vi "GMU2 Calib Shutdown.vi"() -> ()   [LabVIEW 2022 SP3]
uses:
  Traverse_cluster.ctl
  Spacing.ctl
  Controls/Multi_run_mode.ctl
  Controls/User_Specific_mode.ctl
  ADAM Client/Sub VIs/ADAM Controls/Client_Source_Status.ctl
  Controls/GMU Gas Line Name.ctl
panel:
  in  "stop":bool
  out "Purge time (s)":sgl(slide) scale=0.0..600.0
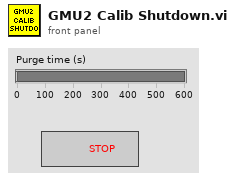
[diagram p1: front panel]
types:
  T1 = typedef "GMU Gas Line Name.ctl" = enum16{"GMU1 Source", "GMU2 Source", "GMU2 Calib", "CPP GRC-A", "CPP GRC-B"}
  T2 = typedef "Client_Source_Status.ctl" = enum16{"Not Using", "Using", "Must Have"}
  T3 = typedef "User_Specific_mode.ctl" = enum16{"Check VI only", "Run VI"}
  T4 = typedef "Traverse_cluster.ctl" = cluster{"Start X":sgl, "Start Y":sgl, "Start Z":sgl, "End X":sgl, "End Y":sgl, "End Z":sgl, "nPoints":i32, "Spacing":T5, "Filename":path, "Tunnel Speed":dbl, "Averaging time (mins)":dbl, "Extra Commands":string, "Carrier_1 Q (l/min)":dbl, "Carrier_2 Q (l/min)":dbl, "Trace Gas Concentration (%)":dbl, "Specific Arguments":string, "Comments":string, "Row No":i32, "Row Type Selector":T6, "EstCompl":string, "Row Duration (mins)":dbl, "nValidPoints":i32, "Meas Setup File":string}
  T5 = typedef "Spacing.ctl" = enum16{"Linear", "Log", "Gauss", "Specified", "N/A"}
  T6 = typedef "Multi_run_mode.ctl" = enum16{"Move Traverse Only", "Set Tunnel Speed Only", "Set Source Only", "Set Measurement Conditions", "Single Measurement", "Vertical Profile", "Lateral Profile", "Longitudinal Profile", "Multi-Axis Profile", "Explore Volume", "Auto Calibrate", "Meas Fast FID Bkgnd", "Check Beam Power", "Scanning Valve Measurement", "Run VI Named:", "Set ADAM Ch", "Wait (minutes)", "Send Message", "Synchronize With:", "Fall Back to this Row", "Turn Off Row Repeating", "Traverse 3D Volume", "Blank Row", "Jump to Fall Back Row"}
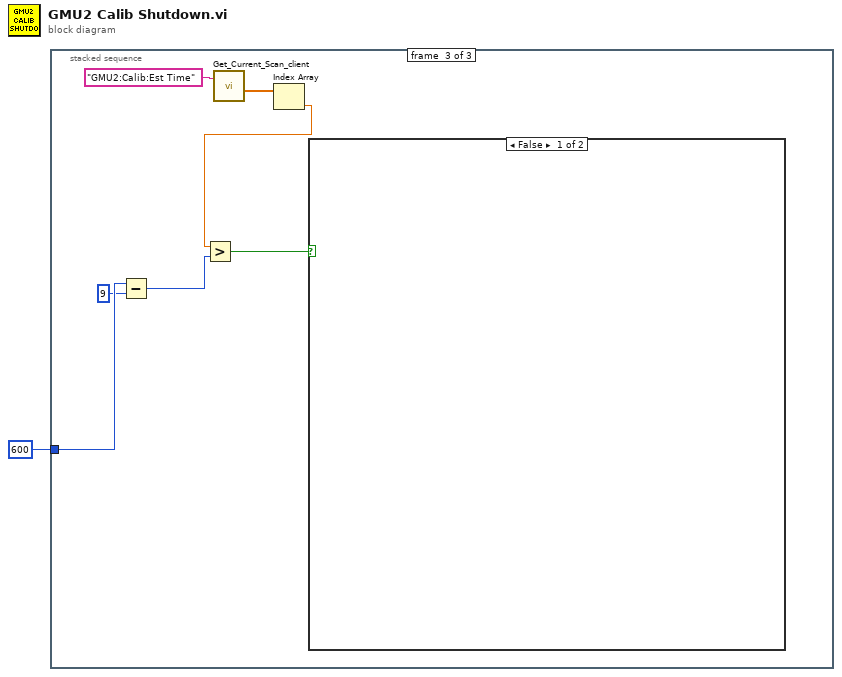
[diagram p0: block diagram]
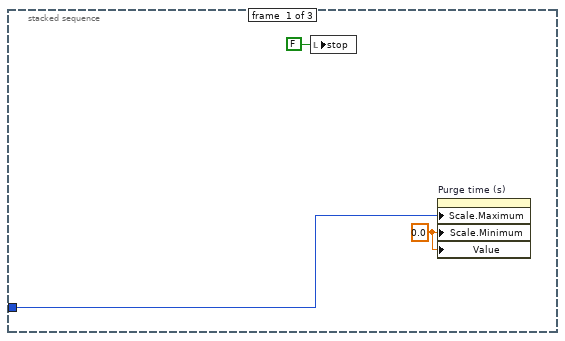
[diagram p2: hidden frame]
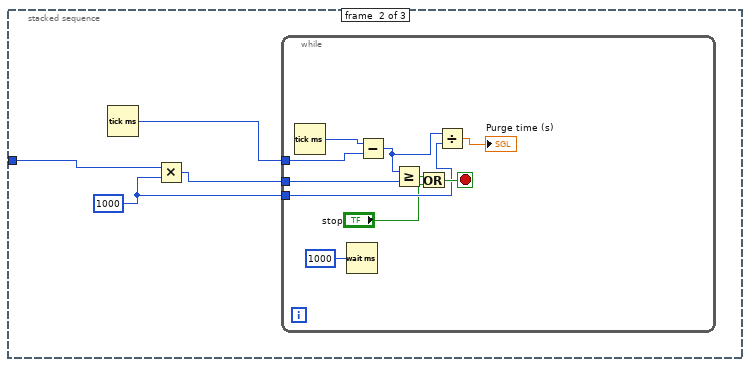
[diagram p3: hidden frame]
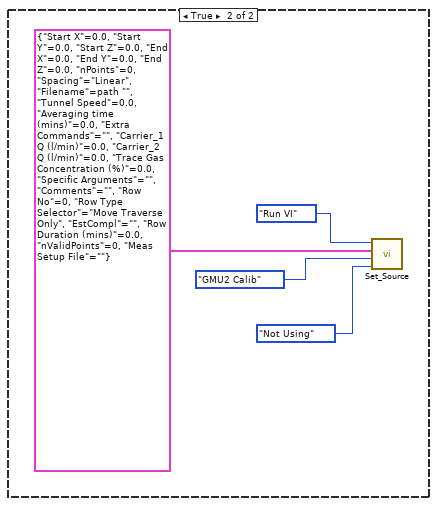
[diagram p4: hidden frame]
diagram:
  n1 = stacked-sequence {
    tunnel: 600 -> [w4 w7 w22]
    frame #0 {
      w3 = 0.0 ("Scale.Range:Minimum")
      n2 = local write "stop"(FALSE ("stop")) -> ()
      n3 = property on="Purge time (s)" class="Slide (strict)"("Scale.Maximum"=w4, "Scale.Minimum"=w3, "Value"=w3) -> ()  [unwired: 2 in, 2 out]
    }
    frame #1 {
      w5 = 1000 ("y")
      n4 = Tick Count (ms)() -> (millisecond timer value=w8:u32)
      n5 = Multiply(x=w7, y=w5) -> (x*y=w6:i32)
      n6 = while {
        tunnel: w6 -> [w17]
        tunnel: w8 -> [w13]
        tunnel: w5 -> [w11]
        stop <- w15 stop-if-true
        n7 = Tick Count (ms)() -> (millisecond timer value=w14:u32)
        n8 = Wait (ms)(milliseconds to wait=u32 1000) -> ()  [unwired: 1 out]
        n9 = Subtract(x=w14, y=w13) -> (x-y=w12:u32)
        n10 = Greater Or Equal?(x=w12, y=w17) -> (x >= y?=w16:bool)
        n11 = Or(x=w16, y="stop") -> (x .or. y?=w15:bool)
        n12 = Divide(x=w12, y=w11) -> (x/y=→"Purge time (s)":dbl)
      }
    }
    frame #2 {
      n13 = Subtract(x=w22, y=9) -> (x-y=w20:i32)
      n14 = call "Get_Current_Scan_client.vi"("singleChannel"="GMU2:Calib:Est Time") -> ("Numerical Values"=w25:dbl[])  [unwired: 1 in, 3 out]
      n15 = Index Array(array=w25) -> (element=w23:dbl)  [unwired: 1 in]
      n16 = Greater?(x=w23, y=w20) -> (0:w19:bool)
      n17 = case shown="False" w19 {
        frame False {
        }
        frame True {
          n18 = call "Set_Source.vi"("Source Status"=Client_Source_Status."Not Using", "Gas Line Name"=GMU_Gas_Line_Name."GMU2 Calib", "Traverse line"=T4 {"Start X"=0.0, "Start Y"=0.0, "Start Z"=0.0, "End X"=0.0, "End Y"=0.0, "End Z"=0.0, "nPoints"=0, "Spacing"=enum."Linear", "Filename"=path "", "Tunnel Speed"=0.0, "Averaging time (mins)"=0.0, "Extra Commands"="", "Carrier_1 Q (l/min)"=0.0, "Carrier_2 Q (l/min)"=0.0, "Trace Gas Concentration (%)"=0.0, "Specific Arguments"="", "Comments"="", "Row No"=0, "Row Type Selector"=enum."Move Traverse Only", "EstCompl"="", "Row Duration (mins)"=0.0, "nValidPoints"=0, "Meas Setup File"=""}, "Simulate/Run"=User_Specific_mode."Run VI") -> ()  [unwired: 1 in, 6 out]
        }
      }
    }
  }
